vi "FormCalibra2.vi"() -> ()   [LabVIEW 2014]
uses:
  testMachine.ctl
  mainMachine.ctl
  <vilib>/Analysis/baseanly.llb/Mean (DBL).vi
  <vilib>/express/express shared/transition.llb/Dynamic To Waveform Array.vi
  <vilib>/express/express signal manip/GetorSetDDTAttributes/Set DDT Attributes/SetT0.vi
  <vilib>/express/express shared/transition.llb/Waveform Array To Dynamic.vi
  <vilib>/express/express signal manip/GetorSetDDTAttributes/Set DDT Attributes/Set DDT Properties.xnode
  <vilib>/Analysis/NI_AALBase.lvlib
panel:
  in  "stop":bool
  out "ledSpeed":bool caption="Velocidade"
  out "error out":errorcluster
  out "ledAcquireState":bool caption="Acquire State"
  out "editTotalLowerLimit":dbl
  out "editCountLowerLimit":dbl
  out "editTotalUpperLimit":dbl
  out "editCountUpperLimit":dbl
  out "ledEnsaio 3":bool
  out "ledBrakeState":bool caption="Brake State"
  out "ledExitState":bool caption="Exit State"
  out "ledMotorState":bool caption="Motor State"
  out "ledInit2State":bool caption="Init State"
  out "ledBlockState":bool caption="Block State"
  out "ledRunningState":bool caption="Running State"
  out "ledReadyState":bool caption="Ready State"
  out "ledInitState":bool caption="Init State"
  out "mainMachine":T1
  out "testMachine":T2=enum."finish"
  in  "editSetPathToFile":path
  out "ledForce":bool caption="Célula de Carga"
  out "ledEngSpeed":bool caption="Rotação"
  out "ledTempB":bool caption="Temperatura B"
  out "ledTempA":bool caption="Temperatura A"
  out "ledTempRef":bool caption="Tempertura (Ref)"
  in  "buttonStop":bool
  in  "buttonStart":bool
  out "graphForce":dynamicdata(graph)
  in  "editOffsetForce":dbl caption="Tara" min=0.0 max=100.0 step=0.1
  in  "editSetForce":dbl caption="Fator de conversão"
  out "editForce":dbl caption="Força (Kgf)" format="%#_4f"
  out "graphSpeed":dynamicdata(graph)
  in  "editSetSpeed":dbl caption="Fator de conversão"
  out "editSpeed":dbl caption="Velocidade (km/h)" format="%#_4f"
  out "editEngineSpeed":dbl caption="Rotação (RPM)" format="%#_4f"
  in  "buttonMotor":bool
  in  "buttonBrake":bool
  in  "editSetWaitLowerTime":u32 caption="Tempo de espera (s)"
  in  "editSetWaitUpperTime":u32 caption="Tempo de espera (s)"
  in  "editSetNumberOfCycles":u32 caption="Número de ciclos" max=999 step=1 format="%0d"
  in  "editSetLowerLimit":u32 caption="Limite inferior (km/h)"
  in  "editSetUpperLimit":u32 caption="Limite superior (km/h)"
  out "editTempB":dbl caption="Temperatura B (ºC)"
  out "editTempA":dbl caption="Temperatura A (ºC)"
  in  "editSetTempRef":dbl caption="Offset referência" step=0.01 format="%#_2f"
  out "editTempRef":dbl caption="Referência (ºC)"
  out "ledMotor":bool
  out "ledBrake":bool
  out "ledEnsaio":bool
  out "labelTotalCycle":string
  out "labelCurrentCycle":string
  out "labelSystemTitle":string
  in  "editCurrCycleCtr":u32
  in  "velocidade 2":u32
  out "velocidade":u32
  # "Bancada de Frenagem - Ensaio"
  # "Sensores"
  # "Temperatura"
  # "Rotação"
  # "Célula de Carga"
  # "Configurações do ensaio"
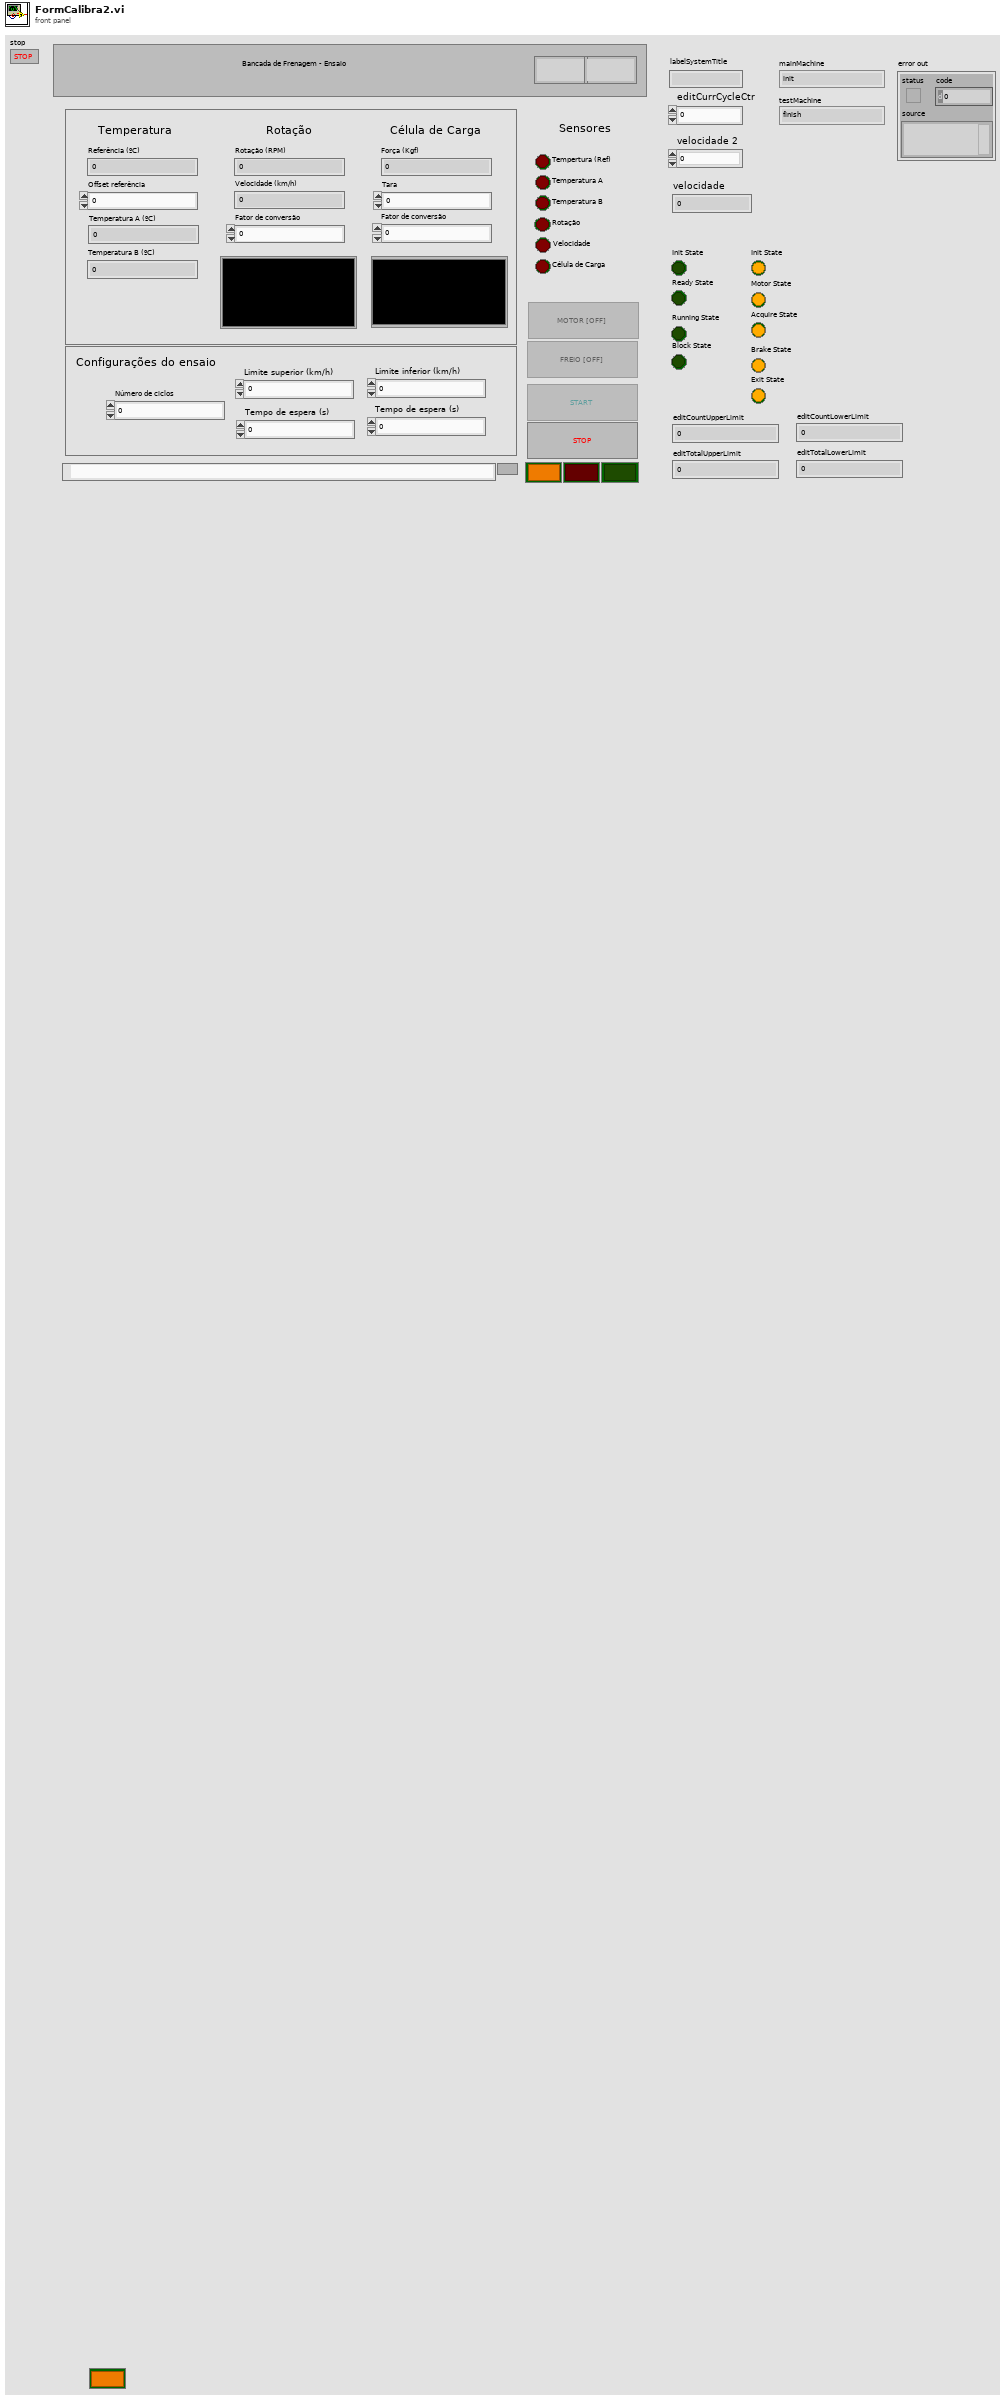
[diagram p1: front panel]
types:
  T1 = typedef "mainMachine.ctl" = enum16{"init", "ready", "running", "blocked", "finish"}
  T2 = typedef "testMachine.ctl" = enum16{"init", "motor", "motor acquire", "brake acquire", "brake", "finish", "exit"}
  T3 = enum8{"Enabled", "Disabled", "Disabled and Grayed Out"}
  T4 = enum16{"Left Button", "Center Button", "Right Button", "Window Close"}
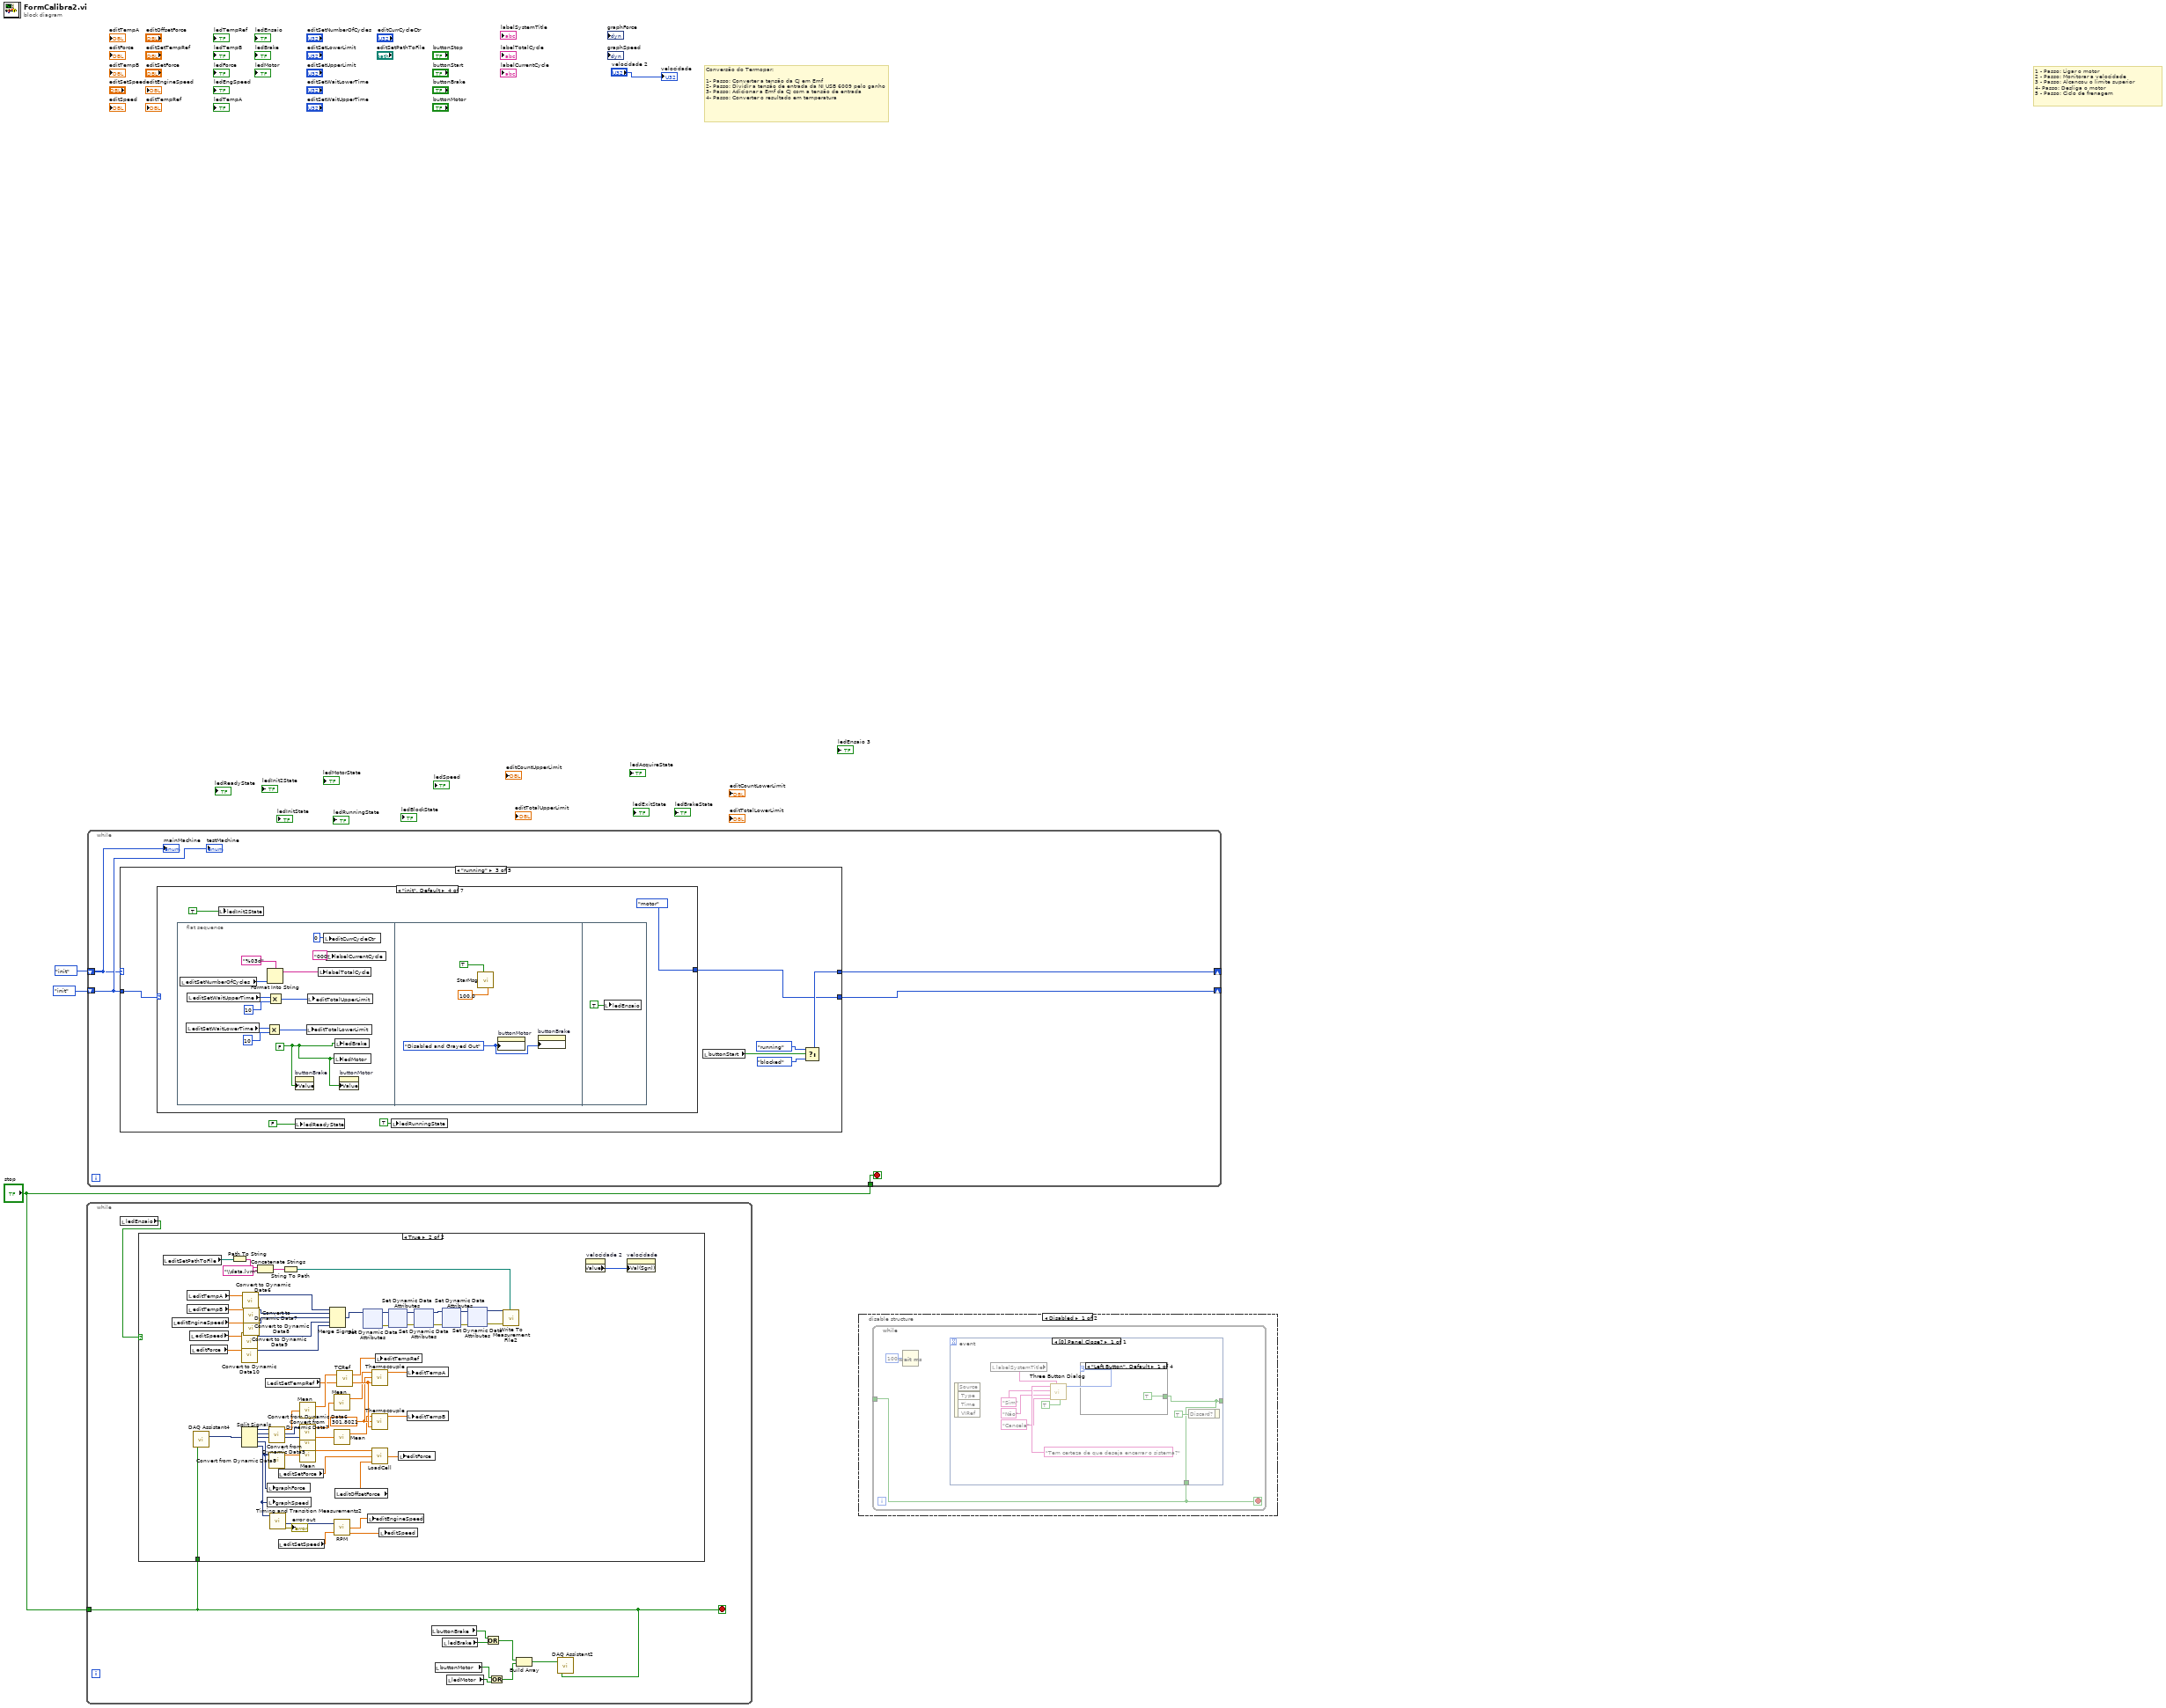
[diagram p0: block diagram]
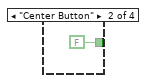
[diagram p2: hidden frame]
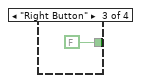
[diagram p3: hidden frame]
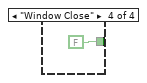
[diagram p4: hidden frame]
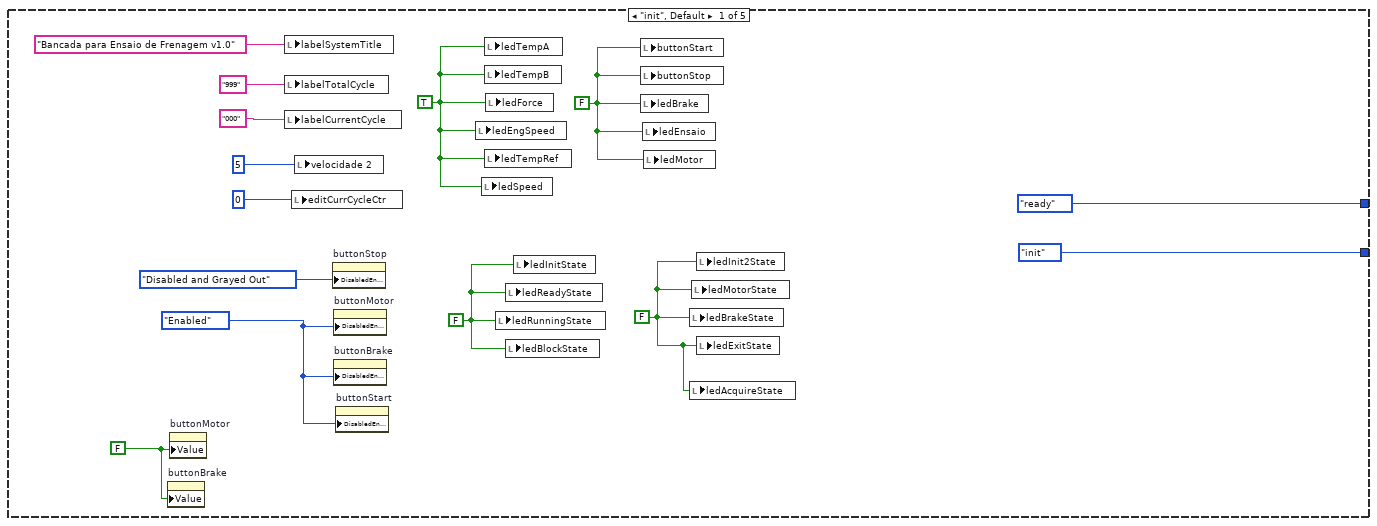
[diagram p7: hidden frame]
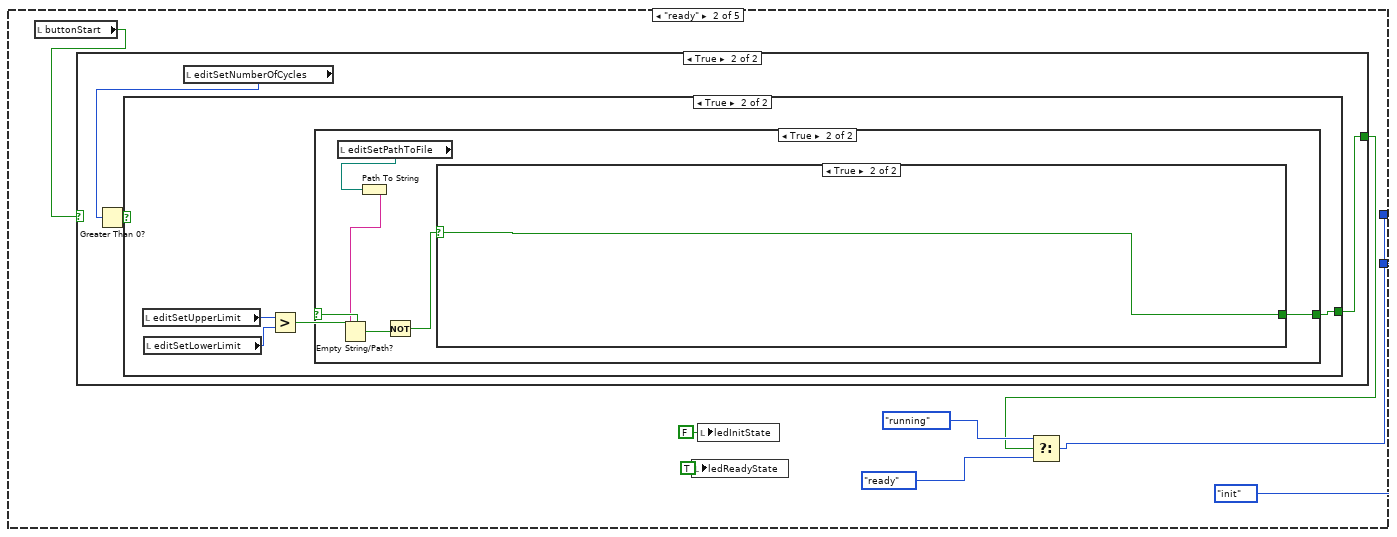
[diagram p8: hidden frame]
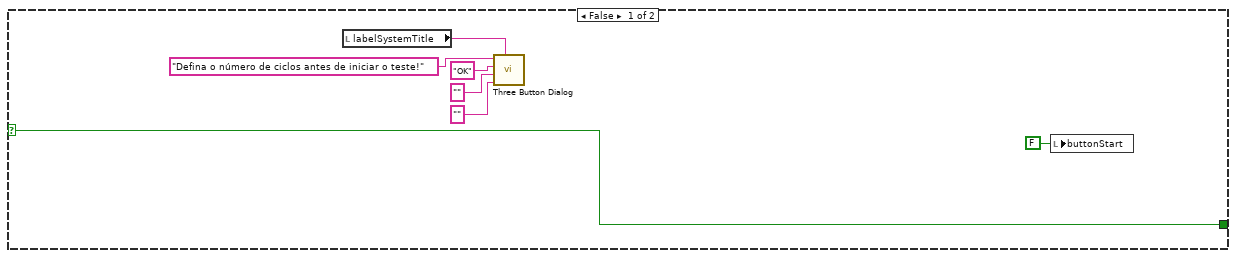
[diagram p10: hidden frame]
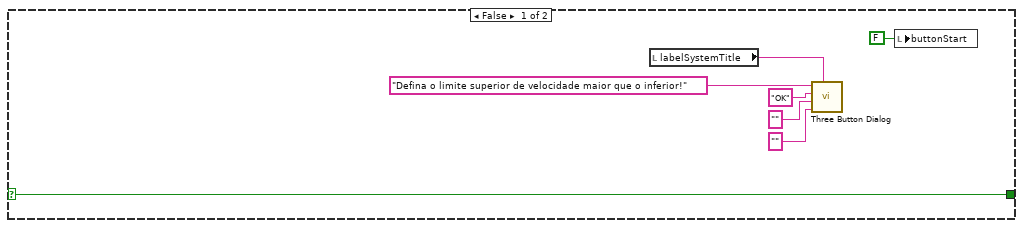
[diagram p11: hidden frame]
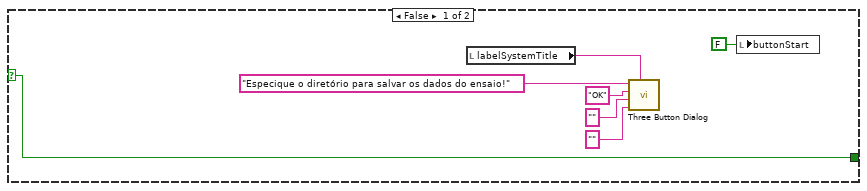
[diagram p12: hidden frame]
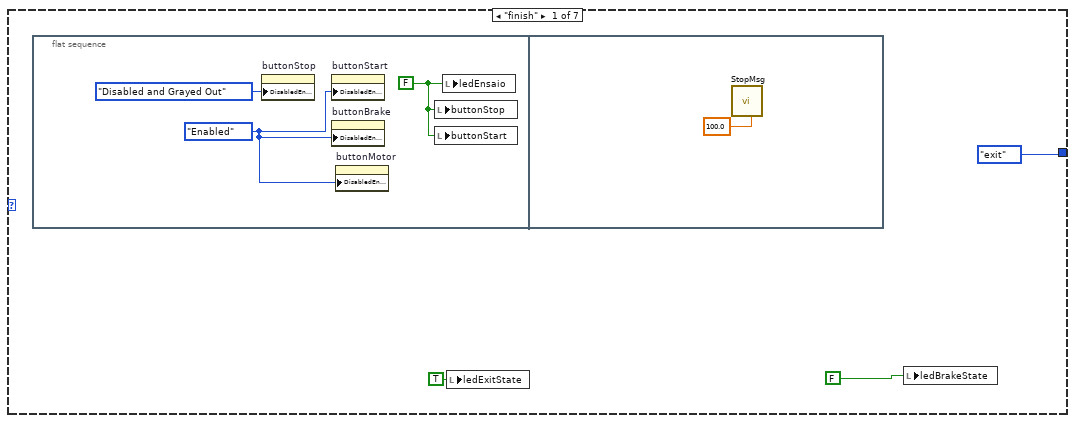
[diagram p13: hidden frame]
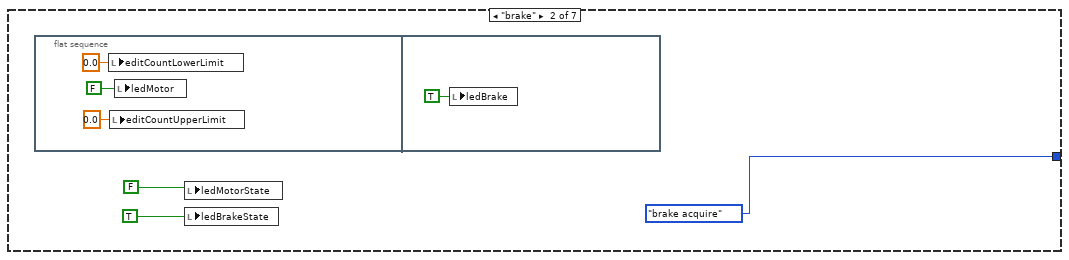
[diagram p14: hidden frame]
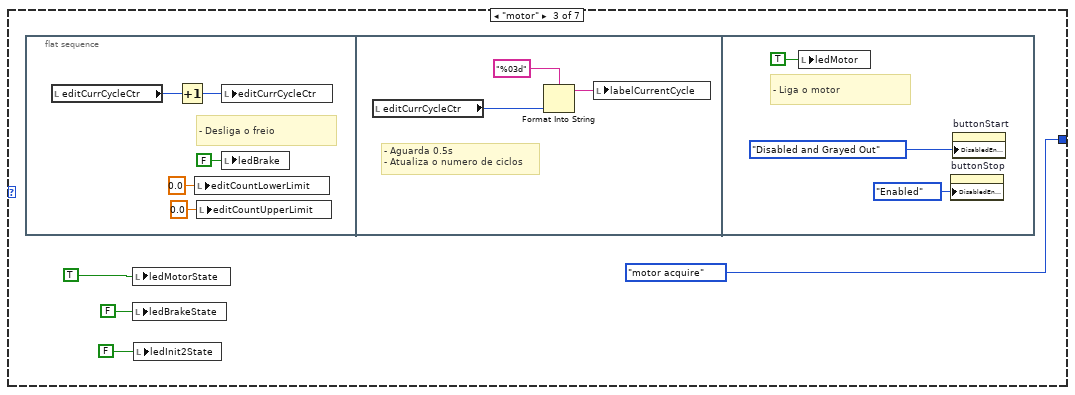
[diagram p15: hidden frame]
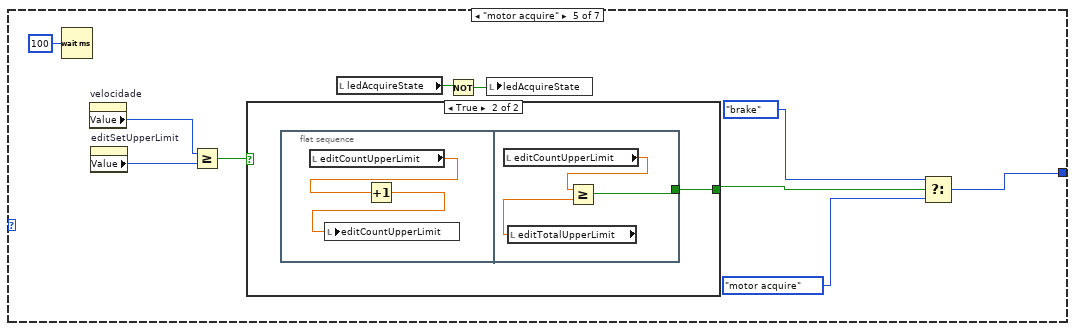
[diagram p16: hidden frame]
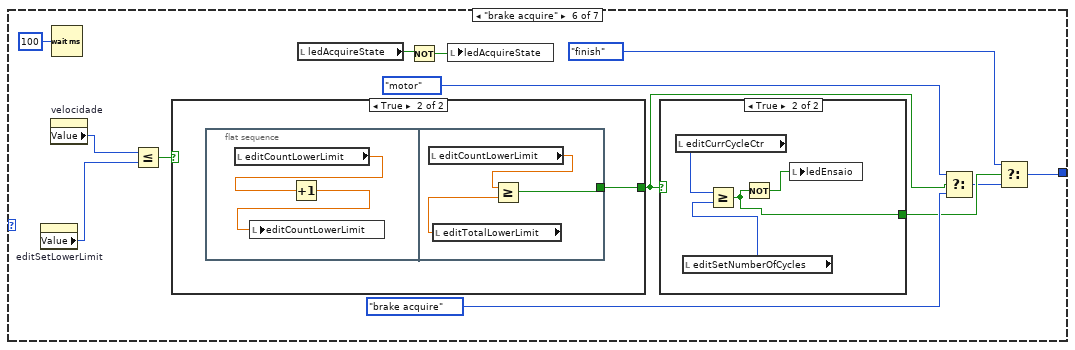
[diagram p18: hidden frame]
diagram:
  # "1 - Passo: Ligar o motor\n2 - Passo: Monitorar a velocidade\n3 - Passo: Alcancou o limite superior\n4- Passo: Desliga o motor\n5 - Passo: Ciclo de frenagem"
  # "Conversão do Termopar:\n\n1- Passo: Converter a tensão da CJ em Emf\n2- Passo: Dividir a tensão de entrada da NI USB 6009 pelo ganho\n3- Passo: Adicionar a Emf da CJ com a tensão de entrada\n4- Passo: Converter o resultado em temperatura"
  n1 = while {
    tunnel: "stop" -> [w5]
    stop <- w5 stop-if-true
    n2 = local read "ledEnsaio"() -> (w13:bool)
    n3 = case shown="True" w13 {
      tunnel: w5 -> [_ w14]
      frame False {
      }
      frame True {
        w27 = 301.8021 ("factor")
        n4 = local read "editSetPathToFile"() -> (w45:path)
        n5 = local read "editEngineSpeed"() -> (w60:dbl)
        n6 = local read "editTempA"() -> (w57:dbl)
        n7 = local read "editTempB"() -> (w59:dbl)
        n8 = local read "editSpeed"() -> (w61:dbl)
        n9 = local read "editForce"() -> (w62:dbl)
        n10 = call "DAQ Assistant4"("stop (F)"=w14) -> ("data"=w16:dynamicdata)  [unwired: 15 in, 3 out]
        n11 = Path To String(path=w45) -> (string=w44:string)
        n12 = call "Convert to Dynamic Data9"("Double"=w61) -> ("Dynamic Data Type"=w65:dynamicdata)  [unwired: 3 in]
        n13 = call "Convert to Dynamic Data10"("Double"=w62) -> ("Dynamic Data Type"=w66:dynamicdata)  [unwired: 3 in]
        n14 = Split Signals(w16) -> (w19:dynamicdata, w23:dynamicdata, w21:dynamicdata, w33:dynamicdata, w32:dynamicdata)  [unwired: 5 in]
        n15 = call "Convert to Dynamic Data6"("Double"=w57) -> ("Dynamic Data Type"=w58:dynamicdata)  [unwired: 3 in]
        n16 = call "Convert to Dynamic Data7"("Double"=w59) -> ("Dynamic Data Type"=w63:dynamicdata)  [unwired: 3 in]
        n17 = call "Convert to Dynamic Data8"("Double"=w60) -> ("Dynamic Data Type"=w64:dynamicdata)  [unwired: 3 in]
        n18 = Concatenate Strings(w44, "\\data.lvm" ("string")) -> (w47:string)
        n19 = local read "editSetTempRef"() -> (w18:dbl)
        n20 = local write "graphForce"(w33) -> ()
        n21 = local write "graphSpeed"(w32) -> ()
        n22 = call "Convert from Dynamic Data5"("Dynamic Data Type"=w19) -> ("Array"=w41:dbl[])  [unwired: 3 in]
        n23 = call "Convert from Dynamic Data8"("Dynamic Data Type"=w33) -> ("Array"=w24:dbl[])  [unwired: 3 in]
        n24 = call "Timing and Transition Measurements2"("Signals"=w32) -> ("error out"=→"error out":errorcluster, "Frequency"=w34:dynamicdata)  [unwired: 9 in]
        n25 = local read "editSetForce"() -> (w39:dbl)
        n26 = local read "editSetSpeed"() -> (w35:dbl)
        n27 = String To Path(string=w47) -> (path=w48:path)
        n28 = call-poly <vilib>:"Mean.vi"("X"=w41) -> ("mean"=w42:dbl)  [unwired: 1 out]
        n29 = call "Convert from Dynamic Data6"("Dynamic Data Type"=w23) -> ("Array"=w20:dbl[])  [unwired: 3 in]
        n30 = call "Convert from Dynamic Data7"("Dynamic Data Type"=w21) -> ("Array"=w22:dbl[])  [unwired: 3 in]
        n31 = call-poly <vilib>:"Mean.vi"("X"=w24) -> ("mean"=w31:dbl)  [unwired: 1 out]
        n32 = Merge Signals(w58, w63, w64, w65, w66) -> (w67:dynamicdata)
        n33 = call-poly <vilib>:"Mean.vi"("X"=w20) -> ("mean"=w25:dbl)  [unwired: 1 out]
        n34 = call-poly <vilib>:"Mean.vi"("X"=w22) -> ("mean"=w26:dbl)  [unwired: 1 out]
        n35 = call "RPM.vi"("data"=w34, "factor"=w35) -> ("RPM"=w37:dbl, "km/h"=w38:dbl)  [unwired: 1 out]
        n36 = local read "editOffsetForce"() -> (w40:dbl)
        n37 = call "TCRef.vi"("offset"=w18, "data"=w42) -> ("emf(mV)"=w28:dbl, "temp (degC)"=w17:dbl)
        n38 = xnode ("Set Dynamic Data Attributes")("Signals In"=w67) -> ("Signals Out"=w49:dynamicdata, "error out"=w51:errorcluster)  [unwired: 4 in]
        n39 = local write "editEngineSpeed"(w37) -> ()
        n40 = call "Thermocouple.vi"("cj(mV)"=w28, "factor"=w27, "data"=w25) -> ("temp(degC)"=w29:dbl)  [unwired: 2 out]
        n41 = call "Thermocouple.vi"("cj(mV)"=w28, "factor"=w27, "data"=w26) -> ("temp(degC)"=w30:dbl)  [unwired: 2 out]
        n42 = call "LoadCell.vi"("tara"=w40, "factor"=w39, "data"=w31) -> ("force (Kgf)"=w36:dbl)
        n43 = local write "editTempRef"(w17) -> ()
        n44 = local write "editSpeed"(w38) -> ()
        n45 = xnode ("Set Dynamic Data Attributes")("Signals In"=w49, "error in"=w51) -> ("Signals Out"=w50:dynamicdata, "error out"=w52:errorcluster)  [unwired: 3 in]
        n46 = local write "editForce"(w36) -> ()
        n47 = local write "editTempA"(w29) -> ()
        n48 = local write "editTempB"(w30) -> ()
        n49 = xnode ("Set Dynamic Data Attributes")("Signals In"=w50, "error in"=w52) -> ("Signals Out"=w68:dynamicdata, "error out"=w53:errorcluster)  [unwired: 3 in]
        n50 = xnode ("Set Dynamic Data Attributes")("Signals In"=w68, "error in"=w53) -> ("Signals Out"=w69:dynamicdata, "error out"=w54:errorcluster)  [unwired: 3 in]
        n51 = xnode ("Set Dynamic Data Attributes")("Signals In"=w69, "error in"=w54) -> ("Signals Out"=w55:dynamicdata, "error out"=w56:errorcluster)  [unwired: 3 in]
        n52 = call "Write To Measurement File2"("Signals"=w55, "error in (no error)"=w56, "Filename"=w48) -> ()  [unwired: 14 in, 3 out]
        n53 = property on="velocidade 2" class="DigNum (strict)"() -> ("Value"=w43:u32)  [unwired: 2 in, 2 out]
        n54 = property on="velocidade" class="DigNum (strict)"("Val(Sgnl)"=w43) -> ()  [unwired: 2 in, 2 out]
      }
    }
    n55 = local read "buttonBrake"() -> (w9:bool)
    n56 = local read "buttonMotor"() -> (w7:bool)
    n57 = local read "ledBrake"() -> (w11:bool)
    n58 = local read "ledMotor"() -> (w8:bool)
    n59 = Or(x=w9, y=w11) -> (x .or. y?=w10:bool)
    n60 = Or(x=w7, y=w8) -> (x .or. y?=w6:bool)
    n61 = Build Array(w10, w6) -> (w12:bool[])
    n62 = call "DAQ Assistant2"("data"=w12, "stop (T)"=w5) -> ()  [unwired: 16 in, 2 out]
  }
  n63 = while {
    shift-right: [w164] -> _
    shift-left: mainMachine."init" ("mainMachine") -> [w161]
    shift-right: [w163] -> _
    shift-left: testMachine."init" ("testMachine") -> [w162]
    tunnel: "stop" -> [w160]
    stop <- w160 stop-if-true
    n64 = case shown="\"running\"" w161 {
      tunnel: [mainMachine."ready" ("mainMachine") w179 w224 w320 mainMachine."finish" ("mainMachine")] -> w164
      tunnel: [testMachine."init" ("testMachine") testMachine."init" ("testMachine") w223 testMachine."init" ("testMachine") testMachine."init" ("testMachine")] -> w163
      tunnel: w162 -> [_ _ w222 _ _]
      frame "init", Default {
        w167 = FALSE ("buttonMotor")
        w170 = FALSE
        w171 = FALSE
        w166 = T3."Enabled" ("Disabled")
        w165 = TRUE
        w175 = FALSE ("motor")
        n65 = property on="buttonBrake" class="Bool (strict)"("Value"=w167) -> ()  [unwired: 2 in, 2 out]
        n66 = property on="buttonMotor" class="Bool (strict)"("Value"=w167) -> ()  [unwired: 2 in, 2 out]
        n67 = local write "labelSystemTitle"("Bancada para Ensaio de Frenagem v1.0" ("systemTitle")) -> ()
        n68 = local write "labelTotalCycle"("999" ("totalCycle")) -> ()
        n69 = local write "labelCurrentCycle"("000" ("currentCycle")) -> ()
        n70 = local write "editCurrCycleCtr"(u32 0 ("currentCycleCtr")) -> ()
        n71 = local write "velocidade 2"(u32 5 ("velocidade 2")) -> ()
        n72 = property on="buttonStop" class="Bool (strict)"("DisabledEnum"=T3."Disabled and Grayed Out" ("Disabled")) -> ()  [unwired: 2 in, 2 out]
        n73 = property on="buttonMotor" class="Bool (strict)"("DisabledEnum"=w166) -> ()  [unwired: 2 in, 2 out]
        n74 = property on="buttonBrake" class="Bool (strict)"("DisabledEnum"=w166) -> ()  [unwired: 2 in, 2 out]
        n75 = property on="buttonStart" class="Bool (strict)"("DisabledEnum"=w166) -> ()  [unwired: 2 in, 2 out]
        n76 = local write "ledEngSpeed"(w165) -> ()
        n77 = local write "ledSpeed"(w165) -> ()
        n78 = local write "ledTempA"(w165) -> ()
        n79 = local write "ledTempB"(w165) -> ()
        n80 = local write "ledTempRef"(w165) -> ()
        n81 = local write "ledForce"(w165) -> ()
        n82 = local write "ledRunningState"(w171) -> ()
        n83 = local write "ledReadyState"(w171) -> ()
        n84 = local write "ledBlockState"(w171) -> ()
        n85 = local write "ledInitState"(w171) -> ()
        n86 = local write "buttonStart"(w175) -> ()
        n87 = local write "buttonStop"(w175) -> ()
        n88 = local write "ledBrake"(w175) -> ()
        n89 = local write "ledEnsaio"(w175) -> ()
        n90 = local write "ledMotor"(w175) -> ()
        n91 = local write "ledBrakeState"(w170) -> ()
        n92 = local write "ledAcquireState"(w170) -> ()
        n93 = local write "ledMotorState"(w170) -> ()
        n94 = local write "ledInit2State"(w170) -> ()
        n95 = local write "ledExitState"(w170) -> ()
      }
      frame "ready" {
        n96 = local read "buttonStart"() -> (w182:bool)
        n97 = case shown="True" w182 {
          selector: w182 -> [w187 _]
          tunnel: [w187 w188] -> w181
          frame False {
          }
          frame True {
            n98 = local read "editSetNumberOfCycles"() -> (w189:u32)
            n99 = Greater Than 0?(x=w189) -> (x > 0?=w190:bool)
            n100 = case shown="True" w190 {
              selector: w190 -> [w197 _]
              tunnel: [w197 w198] -> w188
              frame False {
                n101 = local read "labelSystemTitle"() -> (w192:string)
                n102 = call <vilib>:"Three Button Dialog.vi"("Window Title (\"\")"=w192, "Right Button Text (\"Cancel\")"="" ("Right Button Text (\"Cancel\")"), "Center Button Text (\"No\")"="" ("Center Button Text (\"No\")"), "Left Button Text (\"Yes\")"="OK" ("Left Button Text (\"Yes\")"), "message"="Defina o número de ciclos antes de iniciar o teste!") -> ()  [unwired: 6 in, 1 out]
                n103 = local write "buttonStart"(FALSE ("startButton")) -> ()
              }
              frame True {
                n104 = local read "editSetUpperLimit"() -> (w200:u32)
                n105 = local read "editSetLowerLimit"() -> (w199:u32)
                n106 = Greater?(x=w200, y=w199) -> (0:w201:bool)
                n107 = case shown="True" w201 {
                  selector: w201 -> [w208 _]
                  tunnel: [w208 w211] -> w198
                  frame False {
                    n108 = local read "labelSystemTitle"() -> (w203:string)
                    n109 = call <vilib>:"Three Button Dialog.vi"("Window Title (\"\")"=w203, "Right Button Text (\"Cancel\")"="" ("Right Button Text (\"Cancel\")"), "Center Button Text (\"No\")"="" ("Center Button Text (\"No\")"), "Left Button Text (\"Yes\")"="OK" ("Left Button Text (\"Yes\")"), "message"="Defina o limite superior de velocidade maior que o inferior!") -> ()  [unwired: 6 in, 1 out]
                    n110 = local write "buttonStart"(FALSE ("startButton")) -> ()
                  }
                  frame True {
                    n111 = local read "editSetPathToFile"() -> (w213:path)
                    n112 = Path To String(path=w213) -> (string=w212:string)
                    n113 = Empty String/Path?(string/path=w212) -> (empty?=w210:bool)
                    n114 = Not(x=w210) -> (.not. x?=w209:bool)
                    n115 = case shown="True" w209 {
                      selector: w209 -> [w220 w221]
                      tunnel: [w220 w221] -> w211
                      frame False {
                        n116 = local read "labelSystemTitle"() -> (w215:string)
                        n117 = call <vilib>:"Three Button Dialog.vi"("Window Title (\"\")"=w215, "Right Button Text (\"Cancel\")"="" ("Right Button Text (\"Cancel\")"), "Center Button Text (\"No\")"="" ("Center Button Text (\"No\")"), "Left Button Text (\"Yes\")"="OK" ("Left Button Text (\"Yes\")"), "message"="Especique o diretório para salvar os dados do ensaio!") -> ()  [unwired: 6 in, 1 out]
                        n118 = local write "buttonStart"(FALSE ("startButton")) -> ()
                      }
                      frame True {
                      }
                    }
                  }
                }
              }
            }
          }
        }
        n119 = local write "ledReadyState"(TRUE ("ledReady")) -> ()
        n120 = local write "ledInitState"(FALSE ("ledReady")) -> ()
        n121 = Select(t=mainMachine."running" ("mainMachine"), s=w181, f=mainMachine."ready" ("mainMachine")) -> (s? t:f=w179:T1)
      }
      frame "running" {
        n122 = case shown="\"init\", Default" w222 {
          tunnel: [testMachine."exit" ("testMachine") testMachine."brake acquire" ("testMachine") testMachine."motor acquire" ("testMachine") testMachine."motor" ("testMachine") w277 w299 testMachine."exit" ("testMachine")] -> w223
          frame "finish" {
            n123 = flat-sequence {
              frame #0 {
                w233 = FALSE ("ledReady")
                w234 = T3."Enabled" ("Disabled")
                n124 = property on="buttonStop" class="Bool (strict)"("DisabledEnum"=T3."Disabled and Grayed Out" ("Disabled")) -> ()  [unwired: 2 in, 2 out]
                n125 = property on="buttonStart" class="Bool (strict)"("DisabledEnum"=w234) -> ()  [unwired: 2 in, 2 out]
                n126 = property on="buttonBrake" class="Bool (strict)"("DisabledEnum"=w234) -> ()  [unwired: 2 in, 2 out]
                n127 = property on="buttonMotor" class="Bool (strict)"("DisabledEnum"=w234) -> ()  [unwired: 2 in, 2 out]
                n128 = local write "buttonStop"(w233) -> ()
                n129 = local write "buttonStart"(w233) -> ()
                n130 = local write "ledEnsaio"(w233) -> ()
              }
              frame #1 {
                n131 = call "StopMsg.vi"("Max Value (100)"=100.0) -> ()  [unwired: 8 in, 2 out]
              }
            }
            n132 = local write "ledExitState"(TRUE ("ledReady")) -> ()
            n133 = local write "ledBrakeState"(FALSE ("ledReady")) -> ()
          }
          frame "brake" {
            n134 = flat-sequence {
              frame #0 {
                n135 = local write "editCountLowerLimit"(0.0 ("editCountUpperLimit")) -> ()
                n136 = local write "editCountUpperLimit"(0.0 ("editCountUpperLimit")) -> ()
                n137 = local write "ledMotor"(FALSE ("motor")) -> ()
              }
              frame #1 {
                n138 = local write "ledBrake"(TRUE ("freio")) -> ()
              }
            }
            n139 = local write "ledMotorState"(FALSE ("ledReady")) -> ()
            n140 = local write "ledBrakeState"(TRUE ("ledReady")) -> ()
          }
          frame "motor" {
            n141 = flat-sequence {
              frame #0 {
                # "- Desliga o freio"
                n142 = local read "editCurrCycleCtr"() -> (w251:u32)
                n143 = Increment(x=w251) -> (x+1=w250:u32)
                n144 = local write "editCountLowerLimit"(0.0 ("editCountUpperLimit")) -> ()
                n145 = local write "editCountUpperLimit"(0.0 ("editCountUpperLimit")) -> ()
                n146 = local write "editCurrCycleCtr"(w250) -> ()
                n147 = local write "ledBrake"(FALSE ("freio")) -> ()
              }
              frame #1 {
                # "- Aguarda 0.5s \n- Atualiza o numero de ciclos"
                n148 = local read "editCurrCycleCtr"() -> (w253:u32)
                n149 = Format Into String(format string="%03d", w253) -> (resulting string=w254:string)  [unwired: 2 in, 1 out]
                n150 = local write "labelCurrentCycle"(w254) -> ()
              }
              frame #2 {
                # "- Liga o motor"
                n151 = local write "ledMotor"(TRUE ("motor")) -> ()
                n152 = property on="buttonStop" class="Bool (strict)"("DisabledEnum"=T3."Enabled" ("Disabled")) -> ()  [unwired: 2 in, 2 out]
                n153 = property on="buttonStart" class="Bool (strict)"("DisabledEnum"=T3."Disabled and Grayed Out" ("Disabled")) -> ()  [unwired: 2 in, 2 out]
              }
            }
            n154 = local write "ledMotorState"(TRUE ("ledReady")) -> ()
            n155 = local write "ledBrakeState"(FALSE ("ledReady")) -> ()
            n156 = local write "ledInit2State"(FALSE ("ledReady")) -> ()
          }
          frame "init", Default {
            n157 = flat-sequence {
              frame #0 {
                w261 = FALSE ("ensaio")
                n158 = local read "editSetNumberOfCycles"() -> (w270:u32)
                n159 = local read "editSetWaitLowerTime"() -> (w262:u32)
                n160 = local read "editSetWaitUpperTime"() -> (w267:u32)
                n161 = Multiply(x=w262, y=u32 10) -> (x*y=w264:u32)
                n162 = Format Into String(format string="%03d", w270) -> (resulting string=w271:string)  [unwired: 2 in, 1 out]
                n163 = Multiply(x=w267, y=u32 10) -> (x*y=w265:u32)
                n164 = property on="buttonBrake" class="Bool (strict)"("Value"=w261) -> ()  [unwired: 2 in, 2 out]
                n165 = local write "editTotalLowerLimit"(w264) -> ()
                n166 = local write "editTotalUpperLimit"(w265) -> ()
                n167 = local write "labelTotalCycle"(w271) -> ()
                n168 = local write "editCurrCycleCtr"(u32 0 ("currentCycleCtr")) -> ()
                n169 = local write "labelCurrentCycle"("000" ("currentCycle")) -> ()
                n170 = local write "ledMotor"(w261) -> ()
                n171 = local write "ledBrake"(w261) -> ()
                n172 = property on="buttonMotor" class="Bool (strict)"("Value"=w261) -> ()  [unwired: 2 in, 2 out]
              }
              frame #1 {
                w273 = T3."Disabled and Grayed Out" ("Disabled")
                n173 = call "StarMsg.vi"("Show"=TRUE, "Max Value (100)"=100.0) -> ()  [unwired: 7 in, 2 out]
                n174 = property on="buttonMotor" class="Bool (strict)"("DisabledEnum"=w273) -> ()  [unwired: 2 in, 2 out]
                n175 = property on="buttonBrake" class="Bool (strict)"("DisabledEnum"=w273) -> ()  [unwired: 2 in, 2 out]
              }
              frame #2 {
                n176 = local write "ledEnsaio"(TRUE ("ensaio")) -> ()
              }
            }
            n177 = local write "ledInit2State"(TRUE ("ledReady")) -> ()
          }
          frame "motor acquire" {
            n178 = Wait (ms)(milliseconds to wait=u32 100) -> ()  [unwired: 1 out]
            n179 = property on="velocidade" class="DigNum (strict)"() -> ("Value"=w284:u32)  [unwired: 2 in, 2 out]
            n180 = property on="editSetUpperLimit" class="DigNum (strict)"() -> ("Value"=w285:u32)  [unwired: 2 in, 2 out]
            n181 = Greater Or Equal?(x=w284, y=w285) -> (x >= y?=w281:bool)
            n182 = case shown="True" w281 {
              selector: w281 -> [w287 _]
              tunnel: [w287 w288] -> w280
              frame False {
              }
              frame True {
                n183 = flat-sequence {
                  tunnel: [w291] -> w288
                  frame #0 {
                    n184 = local read "editCountUpperLimit"() -> (w289:dbl)
                    n185 = Increment(x=w289) -> (x+1=w290:dbl)
                    n186 = local write "editCountUpperLimit"(w290) -> ()
                  }
                  frame #1 {
                    n187 = local read "editCountUpperLimit"() -> (w293:dbl)
                    n188 = local read "editTotalUpperLimit"() -> (w292:dbl)
                    n189 = Greater Or Equal?(x=w293, y=w292) -> (x >= y?=w291:bool)
                  }
                }
              }
            }
            n190 = local read "ledAcquireState"() -> (w283:bool)
            n191 = Not(x=w283) -> (.not. x?=w282:bool)
            n192 = local write "ledAcquireState"(w282) -> ()
            n193 = Select(t=testMachine."brake" ("testMachine"), s=w280, f=testMachine."motor acquire" ("testMachine")) -> (s? t:f=w277:T2)
          }
          frame "brake acquire" {
            n194 = property on="editSetLowerLimit" class="DigNum (strict)"() -> ("Value"=w297:u32)  [unwired: 2 in, 2 out]
            n195 = property on="velocidade" class="DigNum (strict)"() -> ("Value"=w298:u32)  [unwired: 2 in, 2 out]
            n196 = Wait (ms)(milliseconds to wait=u32 100) -> ()  [unwired: 1 out]
            n197 = Less Or Equal?(x=w298, y=w297) -> (x <= y?=w303:bool)
            n198 = case shown="True" w303 {
              selector: w303 -> [w312 _]
              tunnel: [w312 w313] -> w301
              frame False {
              }
              frame True {
                n199 = flat-sequence {
                  tunnel: [w316] -> w313
                  frame #0 {
                    n200 = local read "editCountLowerLimit"() -> (w314:dbl)
                    n201 = Increment(x=w314) -> (x+1=w315:dbl)
                    n202 = local write "editCountLowerLimit"(w315) -> ()
                  }
                  frame #1 {
                    n203 = local read "editCountLowerLimit"() -> (w318:dbl)
                    n204 = local read "editTotalLowerLimit"() -> (w317:dbl)
                    n205 = Greater Or Equal?(x=w318, y=w317) -> (x >= y?=w316:bool)
                  }
                }
              }
            }
            n206 = local read "ledAcquireState"() -> (w305:bool)
            n207 = Not(x=w305) -> (.not. x?=w304:bool)
            n208 = local write "ledAcquireState"(w304) -> ()
            n209 = case shown="True" w301 {
              selector: w301 -> [w307 _]
              tunnel: [w307 w309] -> w296
              frame False {
              }
              frame True {
                n210 = local read "editCurrCycleCtr"() -> (w310:u32)
                n211 = local read "editSetNumberOfCycles"() -> (w311:u32)
                n212 = Greater Or Equal?(x=w310, y=w311) -> (x >= y?=w309:bool)
                n213 = Not(x=w309) -> (.not. x?=w308:bool)
                n214 = local write "ledEnsaio"(w308) -> ()
              }
            }
            n215 = Select(t=testMachine."motor" ("testMachine"), s=w301, f=testMachine."brake acquire" ("testMachine")) -> (s? t:f=w295:T2)
            n216 = Select(t=testMachine."finish" ("testMachine"), s=w296, f=w295) -> (s? t:f=w299:T2)
          }
          frame "exit" {
          }
        }
        n217 = local write "ledReadyState"(FALSE ("ledReady")) -> ()
        n218 = local write "ledRunningState"(TRUE ("ledReady")) -> ()
        n219 = local read "buttonStart"() -> (w227:bool)
        n220 = Select(t=mainMachine."running" ("mainMachine"), s=w227, f=mainMachine."blocked" ("mainMachine")) -> (s? t:f=w224:T1)
      }
      frame "blocked" {
        n221 = local read "buttonStart"() -> (w324:bool)
        n222 = Select(t=mainMachine."ready" ("mainMachine"), s=w324, f=mainMachine."blocked" ("mainMachine")) -> (s? t:f=w320:T1)
        n223 = local write "ledRunningState"(FALSE ("ledReady")) -> ()
        n224 = local write "ledBlockState"(TRUE ("ledReady")) -> ()
      }
      frame "finish" {
        n225 = local write "ledBlockState"(FALSE ("ledReady")) -> ()
      }
    }
    "mainMachine" <- w161
    "testMachine" <- w162
  }
  n226 = disable-structure shown="Disabled" {
    frame Disabled {
      n227 = while {
        tunnel: [w331] -> _
        stop <- w331 stop-if-true
        n228 = Wait (ms)(milliseconds to wait=u32 100) -> ()  [unwired: 1 out]
        n229 = event shown="[0] Panel Close?" {
          selector: _ -> [_]
          dyn-events: _ -> [_]
          timeout: _ -> [_]
          tunnel: [w332] -> _
          tunnel: [w332] -> w331
          event Panel Close? {
            n230 = event-data() -> ()  [unwired: 1 in, 4 out]
            n231 = local read "labelSystemTitle"() -> (w336:string)
            n232 = call <vilib>:"Three Button Dialog.vi"("Allow user to close window? (TRUE)"=TRUE, "Window Title (\"\")"=w336, "Right Button Text (\"Cancel\")"="Cancela" ("Right Button Text (\"Cancel\")"), "Center Button Text (\"No\")"="Não" ("Center Button Text (\"No\")"), "Left Button Text (\"Yes\")"="Sim" ("Left Button Text (\"Yes\")"), "message"="Tem certeza de que deseja encerrar o sistema?") -> ("Which Button?"=w337:T4)  [unwired: 5 in]
            n233 = case shown="\"Left Button\", Default" w337 {
              tunnel: [TRUE FALSE FALSE FALSE] -> w332
              frame "Left Button", Default {
              }
              frame "Center Button" {
              }
              frame "Right Button" {
              }
              frame "Window Close" {
              }
            }
            n234 = event-data("Discard?"=TRUE) -> ()  [unwired: 1 in, 1 out]
          }
        }
      }
    }
    frame Enabled {
    }
  }
  "velocidade" <- "velocidade 2"
